vi "Measurement Logic Main.vi"(8 "error in":errorcluster, 9 "measurement configuration":T4={"SERIAL CHANNEL"="SI1", "PATH TO CONFIGURATION SCRIPT"="\"C:\\dev\\scripts\\Image Receiver Scripts\\9296A_RAW8.cpp\"", "REF. CLOCK  (Hz)"=25000000.0, "POC SOURCE"=0, "CSI-2 DATA SOURCE"=0, "SI ACTIVE LANE CNT"=4, "PAYLOAD DATA TYPE"=enum."RAW 8", "INTERPRETATION"=1, "VIRTUAL CHANNEL"=0, "PATTERN"=0, "ALGORITHM"=0, "RIO HANDLER"="PXI1Slot2", "AUTO. VISION DEVICE"=0, "SERIAL (SI) CHANNEL"=1, "BITFILE"="PXIe_1487_4_In_4_Out_Acq_Tap.lvbitx"} {"SERIAL (SI) CHANNEL" items=["SI0", "SI1"]; "AUTO. VISION DEVICE" items=["PXI1Slot2", "PXI1Slot5"]; "ALGORITHM" items=["BILINEAR", "VNG"]; "PATTERN" items=["GB", "GR", "BG", "RG"]; "INTERPRETATION" items=["Grayscale", "Bayer", "RGB", "YUV422", "YUV420", "Legacy YUV420"]; "SI ACTIVE LANE CNT" items=["1 LANE"=1, "2 LANE"=2, "4 LANE"=4]; "CSI-2 DATA SOURCE" items=["CORRECTED", "RAW"]; "POC SOURCE" items=["NONE", "INTERNAL", "AUXILIARY"]}, 10 "measure call context in":refnum<class "Measure Call Context.lvclass">, 11 "user event out":refnum<user-event>) -> (0 "Error Out":errorcluster, 2 "measure call context out":refnum<class "Measure Call Context.lvclass">, 3 "measurement results":T1 {"BYTES ACQUIRED" format="%#.6p"})   [LabVIEW 2025, in "Automotive Vision.lvclass"]
doc: "Contains the core logic for executing the measurement."
uses:
  Automotive Vision.lvclass
  <vilib>/Plug-In SDKs/Measurements/Measure Call Context/Measure Call Context.lvclass
  Measurement Configuration.ctl
  Measurement Results.ctl
  <instrlib>/FlexRIO/CSI-2/v2/Common/Types/LLP Data Type.ctl
  <vilib>/vision/Image Controls.llb/IMAQ Image.ctl
  <instrlib>/FlexRIO/API/Host/v1/NI FlexRIO/API/Wait for PoC Safe to Disconnect Channels Array.vi
  <vilib>/FPGAPlugInAG/Dynamic/niLvFpga_Close_Dynamic.vi
  <extravilib>/ChannelInstances/Event Messenger-bool/Instantiate.vi
  <vilib>/rvi/interface/nirviCloseFPGA/nirviCloseFPGA.xnode
  Automotive Vision.lvclass/Automotive Vision.ctl
  deps/NI148X/Getting Started/Host/Acq/GettingStarted_Acq_148X_Host.lvlib
  deps/NI148X/Getting Started/Host/Common/GettingStarted_Common_148X_Host.lvlib
  <instrlib>/FlexRIO/API/Host/v1/NI FlexRIO API v1.lvlib
  <instrlib>/FlexRIO/CSI-2/v2/Common/NI CSI-2 API Common v2.lvlib
panel:
  in  "Serial Channel (2nd Display)":fxp<+,3,3>
  in  "Serial Channel (1st Display)":fxp<+,3,3>
  in  "Acquired Serial Input Channel Data":T2(tab)
  out "Source Rate (fps)(1st Display)":dbl
  out "Update Rate (fps)(1st Display)":dbl
  out "1st channel display":T3(plugin-control)
  out "Bytes Acquired (1st Channel)":i64 format="%#.6p"
  out "Packets Logged (1st Channel)":i64
  out "Source Rate (fps)(2nd Display)":dbl
  out "Update Rate (fps)(2nd Display)":dbl
  out "2nd channel display":T3(plugin-control)
  out "Packets Logged (2nd Channel)":i64
  out "Bytes Acquired (2nd Channel)":i64 format="%#.6p"
  out "Acquisition In Progress":bool
  out "Acquisition Duration (s)":dbl format="%.1f"
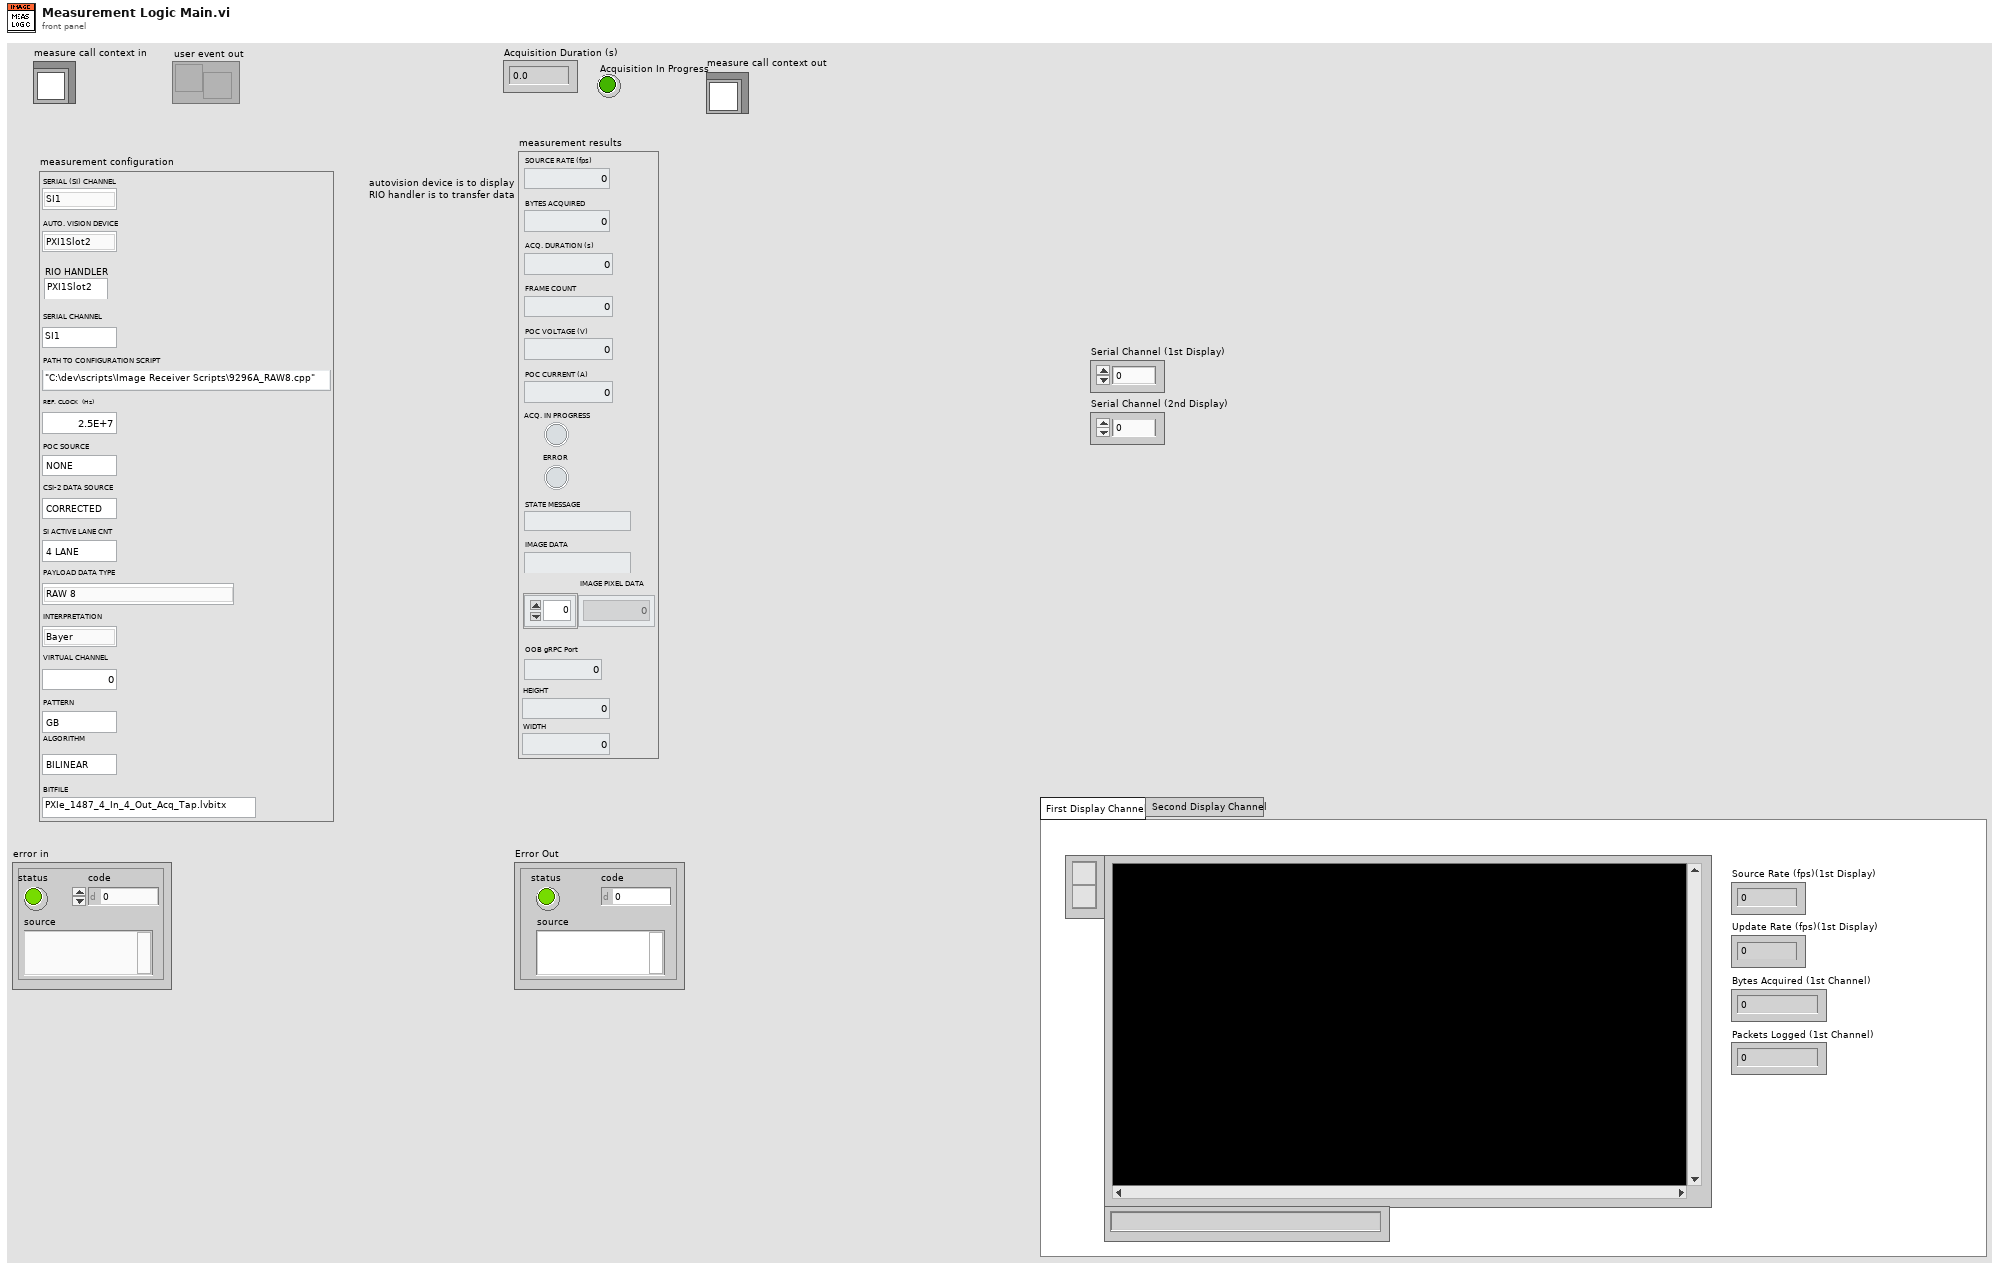
[diagram p1: front panel]
types:
  T1 = typedef "Automotive Vision.lvclass/Measurement Results.ctl" = cluster{"ACQ. IN PROGRESS":bool, "IMAGE PIXEL DATA":u32[], "ACQ. DURATION (s)":dbl, "SOURCE RATE (fps)":dbl, "BYTES ACQUIRED":u64, "FRAME COUNT":u64, "POC VOLTAGE (V)":dbl, "POC CURRENT (A)":dbl, "ERROR":bool, "STATE MESSAGE":string, "IMAGE DATA":string, "OOB gRPC Port":i32, "HEIGHT":u64, "WIDTH":u64}
  T2 = enum32{"First Display Channel", "Second Display Channel"}
  T3 = typedef "IMAQ Image.ctl" = refnum<image>
  T4 = typedef "Automotive Vision.lvclass/Measurement Configuration.ctl" = cluster{"SERIAL CHANNEL":string, "PATH TO CONFIGURATION SCRIPT":string, "REF. CLOCK  (Hz)":dbl, "POC SOURCE":u32, "CSI-2 DATA SOURCE":u32, "SI ACTIVE LANE CNT":u32, "PAYLOAD DATA TYPE":enum32{"Frame Start", "Frame End", "Line Start", "Line End", "End of Transmission", "Reserved 0", "Reserved 1", "Reserved 2", "Generic Short Packet 1", "Generic Short Packet 2", "Generic Short Packet 3", "Generic Short Packet 4", "Generic Short Packet 5", "Generic Short Packet 6", "Generic Short Packet 7", "Generic Short Packet 8", "Null", "Blanking Data", "Embedded 8-bit non Image Data", "Generic Long Packet 1", "Generic Long Packet 2", "Generic Long Packet 3", "Generic Long Packet 4", "Reserved 3", "YUV420 8-bit", "YUV420 10-bit", "Legacy YUV420 8-bit", "Reserved 4", "YUV420 8-bit Chroma Shifted", "YUV420 10-bit Chroma Shifted", "YUV422 8-bit", "YUV422 10-bit", "RGB444", "RGB555", "RGB565", "RGB666", "RGB888", "Reserved 5", "Reserved 6", "RAW 24", "RAW 6", "RAW 7", "RAW 8", "RAW 10", "RAW 12", "RAW 14", "RAW 16", "RAW 20", "User Defined 8-bit Data 1", "User Defined 8-bit Data 2", "User Defined 8-bit Data 3", "User Defined 8-bit Data 4", "User Defined 8-bit Data 5", "User Defined 8-bit Data 6", "User Defined 8-bit Data 7", "User Defined 8-bit Data 8", "USL Command", "Reserved 7", "Reserved 8", "Reserved 9", "Reserved 10", "Reserved 11", "Reserved 12", "LRTE EPD Spacer"}, "INTERPRETATION":u32, "VIRTUAL CHANNEL":u32, "PATTERN":u32, "ALGORITHM":u32, "RIO HANDLER":string, "AUTO. VISION DEVICE":u32, "SERIAL (SI) CHANNEL":u32, "BITFILE":string}
  T5 = typedef "NI CSI-2 API Common v2.lvlib/LLP Data Type.ctl" = enum8{"Frame Start", "Frame End", "Line Start", "Line End", "End of Transmission", "Reserved 0", "Reserved 1", "Reserved 2", "Generic Short Packet 1", "Generic Short Packet 2", "Generic Short Packet 3", "Generic Short Packet 4", "Generic Short Packet 5", "Generic Short Packet 6", "Generic Short Packet 7", "Generic Short Packet 8", "Null", "Blanking Data", "Embedded 8-bit non Image Data", "Generic Long Packet 1", "Generic Long Packet 2", "Generic Long Packet 3", "Generic Long Packet 4", "Reserved 3", "YUV420 8-bit", "YUV420 10-bit", "Legacy YUV420 8-bit", "Reserved 4", "YUV420 8-bit Chroma Shifted", "YUV420 10-bit Chroma Shifted", "YUV422 8-bit", "YUV422 10-bit", "RGB444", "RGB555", "RGB565", "RGB666", "RGB888", "Reserved 5", "Reserved 6", "RAW 24", "RAW 6", "RAW 7", "RAW 8", "RAW 10", "RAW 12", "RAW 14", "RAW 16", "RAW 20", "User Defined 8-bit Data 1", "User Defined 8-bit Data 2", "User Defined 8-bit Data 3", "User Defined 8-bit Data 4", "User Defined 8-bit Data 5", "User Defined 8-bit Data 6", "User Defined 8-bit Data 7", "User Defined 8-bit Data 8", "USL Command", "Reserved 7", "Reserved 8", "Reserved 9", "Reserved 10", "Reserved 11", "Reserved 12", "LRTE EPD Spacer"}
  T6 = typedef "GettingStarted_Common_148X_Host.lvlib/Serial Channel Configuration.ctl" = cluster{"Serial Channel":string, "FPGA Display Parameters":T7, "RAW Display Parameters":cluster{"Interpretation":T8, "Bayer Parameters":cluster{"Pattern":i32, "Algorithm":i32, "Red Gain":dbl, "Green Gain":dbl, "Blue Gain":dbl}}}
  T7 = typedef "NI CSI-2 API FPGA v2.lvlib/Display Parameters.ctl" = cluster{"virtual channel":fxp<+,4,4>, "payload data type":T5, "frame skip count":u16, "line skip count":u8, "pixel skip count":fxp<+,5,5>}
  T8 = typedef "GettingStarted_Common_148X_Host.lvlib/RAW Interpretation for Display.ctl" = enum16{"Grayscale", "Bayer", "RGB", "YUV422", "YUV420", "Legacy YUV420"}
  T9 = typedef "GettingStarted_Common_148X_Host.lvlib/Serial Channel Display Parameters.ctl" = cluster{"images":cluster{"grayscale":T3, "color":T3}, "RAW parameters":cluster{"interpretation":T8, "bayer parameters":cluster{"pattern":i32, "algorithm":i32, "red gain":dbl, "green gain":dbl, "blue gain":dbl}}}
  T10 = cluster{"Acquisition In Progress":refnum<vi>, "Acquisition Duration (s)":refnum<vi>, "Bytes Acquired (1st Channel)":refnum<vi>}
  T11 = typedef "Event Messenger-bool.lvlib/))Channel.ctl" = refnum<queue>
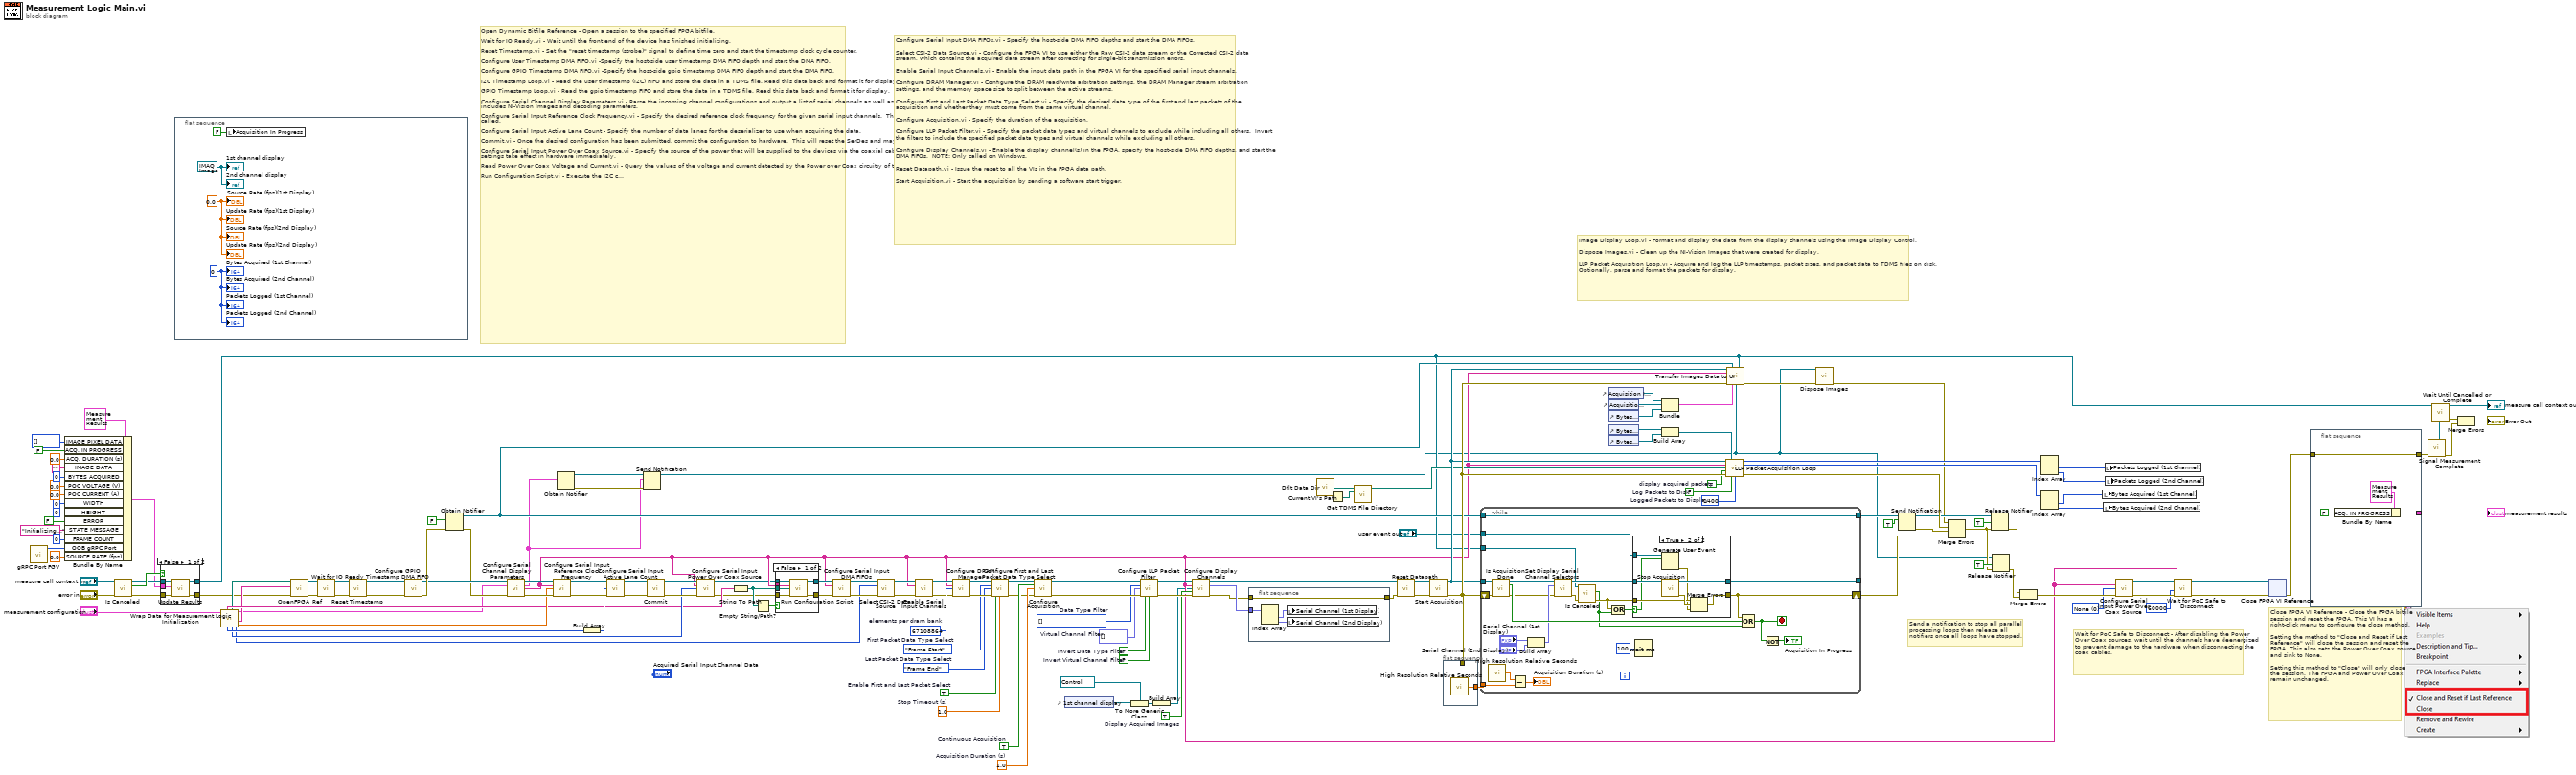
[diagram p0: block diagram]
diagram:
  w77 = i64 1400  # Logged Packets to Display
  w101 = FALSE  # Log Packets to Disk
  w131 = FALSE  # Invert Virtual Channel Filter
  w132 = FALSE  # Invert Data Type Filter
  w133 = fxp<+,4,4>[] []  # Virtual Channel Filter
  w97 = TRUE  # Display Acquired Images
  w135 = T5[] [] items=["Frame Start", "Frame End", "Line Start", "Line End", "End of Transmission", "Reserved 0", "Reserved 1", "Reserved 2", "Generic Short Packet 1", "Generic Short Packet 2", "Generic Short Packet 3", "Generic Short Packet 4", "Generic Short Packet 5", "Generic Short Packet 6", "Generic Short Packet 7", "Generic Short Packet 8", "Null", "Blanking Data", "Embedded 8-bit non Image Data", "Generic Long Packet 1", "Generic Long Packet 2", "Generic Long Packet 3", "Generic Long Packet 4", "Reserved 3", "YUV420 8-bit", "YUV420 10-bit", "Legacy YUV420 8-bit", "Reserved 4", "YUV420 8-bit Chroma Shifted", "YUV420 10-bit Chroma Shifted", "YUV422 8-bit", "YUV422 10-bit", "RGB444", "RGB555", "RGB565", "RGB666", "RGB888", "Reserved 5", "Reserved 6", "RAW 24", "RAW 6", "RAW 7", "RAW 8", "RAW 10", "RAW 12", "RAW 14", "RAW 16", "RAW 20", "User Defined 8-bit Data 1", "User Defined 8-bit Data 2", "User Defined 8-bit Data 3", "User Defined 8-bit Data 4", "User Defined 8-bit Data 5", "User Defined 8-bit Data 6", "User Defined 8-bit Data 7", "User Defined 8-bit Data 8", "USL Command", "Reserved 7", "Reserved 8", "Reserved 9", "Reserved 10", "Reserved 11", "Reserved 12", "LRTE EPD Spacer"]  # Data Type Filter
  w138 = 1.0  # Acquisition Duration (s)
  w141 = TRUE  # Continuous Acquisition
  w121 = 1.0  # Stop Timeout (s)
  w122 = TRUE  # Enable First and Last Packet Select
  w119 = LLP_Data_Type."Frame End"  # Last Packet Data Type Select
  w120 = LLP_Data_Type."Frame Start"  # First Packet Data Type Select
  w58 = 0 items=["None", "Internal", "Auxiliary"] ("power over coax source")
  w78 = TRUE  # display acquired packets
  w147 = u32 67108864  # elements per dram bank
  # "Wait for PoC Safe to Disconnect - After disabling the Power Over Coax sources, wait until the channels have deenergized to prevent damage to the hardware when disconnecting the coax cables."
  # "Send a notification to stop all parallel processing loops then release all notifiers once all loops have stopped."
  # "Image Display Loop.vi - Format and display the data from the display channels using the Image Display Control.   \n\nDispose Images.vi - Clean up the NI-Vision Images that were created for display.\n\nLLP Packet Acquisition Loop.vi - Acquire and log the LLP timestamps, packet sizes, and packet data to TDMS files on disk.  Optionally, parse and format the packets for display."
  # "Configure Serial Input DMA FIFOs.vi - Specify the host-side DMA FIFO depths and start the DMA FIFOs.\n\nSelect CSI-2 Data Source.vi - Configure the FPGA VI to use either the Raw CSI-2 data stream or the Corrected CSI-2 data stream, which contains the acquired data stream after correcting for single-bit transmission errors.\n\nEnable Serial Input Channels.vi - Enable the input data path in the FPGA VI for the specified serial input channels.\n\nConfigure DRAM Manager.vi - Configure the DRAM read/write arbitration settings, the DRAM Manager stream arbitration settings, and the memory space size to split between the active streams.\n\nConfigure First and Last Packet Data Type Select.vi - Specify the desired data type of the first and last packets of the acquisition and whether they must come from the same virtual channel.\n\nConfigure Acquisition.vi - Specify the duration of the acquisition.\n\nConfigure LLP Packet Filter.vi - Specify the packet data types and virtual channels to exclude while including all others.  Invert the filters to include the specified packet data types and virtual channels while excluding all others.\n\nConfigure Display Channels.vi - Enable the display channel(s) in the FPGA, specify the host-side DMA FIFO depths, and start the DMA FIFOs.  NOTE: Only called on Windows. \n\nReset Datapath.vi - Issue the reset to all the VIs in the FPGA data path.\n\nStart Acquisition.vi - Start the acquisition by sending a software start trigger."
  # "Close FPGA VI Reference - Close the FPGA bitfile session and reset the FPGA. This VI has a right-click menu to configure the close method. \n\nSetting the method to \"Close and Reset if Last Reference\" will close the session and reset the FPGA. This also sets the Power Over Coax source and sink to None.\n\nSetting this method to \"Close\" will only close the session. The FPGA and Power Over Coax remain unchanged."
  # "Open Dynamic Bitfile Reference - Open a session to the specified FPGA bitfile.\n\nWait for IO Ready.vi - Wait until the front end of the device has finished initializing.\n\nReset Timestamp.vi - Set the \"reset timestamp (strobe)\" signal to define time zero and start the timestamp clock cycle counter.\n\nConfigure User Timestamp DMA FIFO.vi -Specify the host-side user timestamp DMA FIFO depth and start the DMA FIFO.\n\nConfigure GPIO Timestamp DMA FIFO.vi -Specify the host-side gpio timestamp DMA FIFO depth and start the DMA FIFO.\n\nI2C Timestamp Loop.vi - Read the user timestamp (I2C) FIFO and store the data in a TDMS file. Read this data back and format it for display.\n\nGPIO Timestamp Loop.vi - Read the gpio timestamp FIFO and store the data in a TDMS file. Read this data back and format it for display.\n\nConfigure Serial Channel Display Parameters.vi - Parse the incoming channel configurations and output a list of serial channels as well as a list of serial channel display parameters, which includes NI-Vision Images and decoding parameters.\n\nConfigure Serial Input Reference Clock Frequency.vi - Specify the desired reference clock frequency for the given serial input channels.  These settings do not take effect until Commit.vi is called.\n\nConfigure Serial Input Active Lane Count - Specify the number of data lanes for the deserializer to use when acquiring the data. \n\nCommit.vi - Once the desired configuration has been submitted, commit the configuration to hardware.  This will reset the SerDes and may cause GPIO lines to toggle. \n\nConfigure Serial Input Power Over Coax Source.vi - Specify the source of the power that will be supplied to the devices via the coaxial cables attached to the given serial input channels.  These settings take effect in hardware immediately.\n\nRead Power Over Coax Voltage and Current.vi - Query the values of the voltage and current detected by the Power over Coax circuitry of the given serial channels.\n\nRun Configuration Script.vi - Execute the I2C commands in the specified script file for the given serial channels.  The script is used to configure the serializer, deserializer, or other I2C slave device, such as the image sensor."
  n1 = call "gRPC Port FGV.vi"() -> ("Listening Port out"=w28:i32)  [unwired: 11 in]
  n2 = Bundle By Name(cluster=T1 {"ACQ. IN PROGRESS"=FALSE, "IMAGE PIXEL DATA"=[], "ACQ. DURATION (s)"=0.0, "SOURCE RATE (fps)"=0.0, "BYTES ACQUIRED"=0, "FRAME COUNT"=0, "POC VOLTAGE (V)"=0.0, "POC CURRENT (A)"=0.0, "ERROR"=FALSE, "STATE MESSAGE"="", "IMAGE DATA"="", "OOB gRPC Port"=0, "HEIGHT"=0, "WIDTH"=0} ("Measurement Results"), "IMAGE PIXEL DATA"=u32[] [], "ACQ. IN PROGRESS"=FALSE, "ACQ. DURATION (s)"=0.0, "IMAGE DATA"="", "BYTES ACQUIRED"=u64 0, "POC VOLTAGE (V)"=0.0, "POC CURRENT (A)"=0.0, "WIDTH"=u64 0, "HEIGHT"=u64 0, "ERROR"=FALSE, "STATE MESSAGE"="Initializing...", "FRAME COUNT"=u64 0, "OOB gRPC Port"=w28, "SOURCE RATE (fps)"=0.0) -> (w24:T1)
  n3 = call <vilib>:"Is Canceled.vi"("error in"="error in", "measure call context in"="measure call context in") -> ("error out"=w27:errorcluster, "is canceled?"=w26:bool, "measure call context out"=w25:refnum<class "Measure Call Context.lvclass">)  [unwired: 7 in]
  n4 = case shown="False" w26 {
    tunnel: w24 -> [w156 _]
    tunnel: [w155 w158] -> w21
    tunnel: w25 -> [w154 w157]
    tunnel: w27 -> [w153 w158]
    tunnel: [w152 w157] -> w6
    frame False {
      n5 = call <vilib>:"Update Results.vi"("error in"=w153, "measurement results"=w156, "measure call context in"=w154) -> ("error out"=w155:errorcluster, "measure call context out"=w152:refnum<class "Measure Call Context.lvclass">)  [unwired: 7 in]
    }
    frame True {
    }
  }
  n6 = flat-sequence {
    frame #0 {
      w160 = i64 0 ("Number of Packets Acquired (1st Channel)")
      w161 = 0.0 ("display fps (2nd display)")
      w162 = T3 refnum ("first channel display")
      n7 = local write "Acquisition In Progress"(FALSE ("Acquisition In Progress")) -> ()
      "1st channel display" <- w162
      "2nd channel display" <- w162
      "Update Rate (fps)(1st Display)" <- w161
      "Update Rate (fps)(2nd Display)" <- w161
      "Packets Logged (1st Channel)" <- w160
      "Packets Logged (2nd Channel)" <- w160
      "Source Rate (fps)(1st Display)" <- w161
      "Source Rate (fps)(2nd Display)" <- w161
      "Bytes Acquired (1st Channel)" <- w160
      "Bytes Acquired (2nd Channel)" <- w160
    }
  }
  n8 = call "Wrap Data for Measurement Logic Initialization.vi"("measurement configuration"="measurement configuration") -> ("REF. CLOCK  (Hz)"=w47:dbl, "RIO HANDLER"=w43:string, "CSI-2 DATA SOURCE"=w48:u32, "Serial Input Configuration"=w36:T6[], "POC SOURCE"=w49:u32, "appended path"=w42:path, "SI ACTIVE LANE CNT"=w50:u32, "PATH TO CONFIGURATION SCRIPT"=w46:string)  [unwired: 3 in]
  n9 = call "OpenFPGA_Ref.vi"("error in"=w21, "RIO HANDLER"=w43, "Bitfile path"=w42) -> ("error out"=w37:errorcluster, "Refnum out"=w134:refnum<k20>)  [unwired: 7 in]
  n10 = call <instrlib>:"Wait for IO Ready.vi"("fpga interface in"=w134, "error in"=w37) -> ("fpga interface out"=w94:refnum<k20>, "error out"=w95:errorcluster)  [unwired: 10 in, 2 out]
  n11 = call "Reset Timestamp.vi"("fpga interface in"=w94, "error in (no error)"=w95) -> ("fpga interface out"=w2:refnum<k20>, "error out"=w1:errorcluster)  [unwired: 12 in]
  n12 = call "Configure GPIO Timestamp DMA FIFO.vi"("fpga interface in"=w2, "error in (no error)"=w1) -> ("fpga interface out"=w82:refnum<k20>, "error out"=w84:errorcluster)  [unwired: 12 in]
  n13 = Obtain Notifier(notification data type=FALSE ("result"), error in (no error)=w84) -> (notifier out=w70:refnum<notifier>, error out=w81:errorcluster)  [unwired: 2 in, 1 out]
  n14 = call "Configure Serial Channel Display Parameters.vi"("fpga interface in"=w82, "serial channel configurations"=w36, "error in (no error)"=w81) -> ("fpga interface out"=w111:refnum<k20>, "serial channel display parameters"=w67:T9[], "serial channels"=w35:string[], "error out"=w110:errorcluster)  [unwired: 9 in]
  n15 = call "Configure Serial Input Reference Clock Frequency.vi"("fpga interface in"=w111, "serial input channels"=w35, "serial input reference clock frequency (Hz)"=w47, "error in (no error)"=w110) -> ("fpga interface out"=w75:refnum<k20>, "error out"=w74:errorcluster)  [unwired: 10 in]
  n16 = Obtain Notifier(notification data type=w67) -> (notifier out=w69:refnum<notifier>, error out=w68:errorcluster)  [unwired: 3 in, 1 out]
  n17 = Build Array(w50) -> (w71:u32[])
  n18 = call "Configure Serial Input Active Lane Count.vi"("fpga interface in"=w75, "serial input active lane counts"=w71, "error in (no error)"=w74) -> ("fpga interface out"=w73:refnum<k20>, "error out"=w72:errorcluster)  [unwired: 11 in]
  n19 = Send Notification(notification=w67, notifier=w69, error in (no error)=w68) -> (notifier out=w5:refnum<notifier>)  [unwired: 1 out]
  n20 = call <instrlib>:"Commit.vi"("fpga interface in"=w73, "error in"=w72) -> ("fpga interface out"=w136:refnum<k20>, "error out"=w137:errorcluster)  [unwired: 12 in]
  n21 = call "Configure Serial Input Power Over Coax Source.vi"("fpga interface in"=w136, "serial input channels"=w35, "power over coax source"=w49, "error in (no error)"=w137) -> ("fpga interface out"=w30:refnum<k20>, "error out"=w29:errorcluster)  [unwired: 9 in, 1 out]
  n22 = String To Path(string=w46) -> (path=w45:path)
  n23 = Empty String/Path?(string/path=w45) -> (empty?=w96:bool)
  n24 = case shown="False" w96 {
    tunnel: [w168 w169] -> w145
    tunnel: [w167 w170] -> w140
    tunnel: w29 -> [w166 w169]
    tunnel: w30 -> [w165 w170]
    tunnel: w35 -> [w164 _]
    tunnel: w45 -> [w163 _]
    frame False {
      n25 = call "Run Configuration Script.vi"("fpga interface in"=w165, "serial channels"=w164, "configuration script"=w163, "error in (no error)"=w166) -> ("fpga interface out"=w167:refnum<k20>, "error out"=w168:errorcluster)  [unwired: 10 in]
    }
    frame True {
    }
  }
  n26 = call "Configure Serial Input DMA FIFOs.vi"("fpga interface in"=w140, "serial channels"=w35, "error in (no error)"=w145) -> ("fpga interface out"=w130:refnum<k20>, "error out"=w127:errorcluster)  [unwired: 11 in]
  n27 = call "Select CSI-2 Data Source.vi"("fpga interface in"=w130, "csi-2 data source"=w48, "error in (no error)"=w127) -> ("fpga interface out"=w129:refnum<k20>, "error out"=w128:errorcluster)  [unwired: 11 in]
  n28 = call "Enable Serial Input Channels.vi"("fpga interface in"=w129, "serial input channels"=w35, "error in (no error)"=w128) -> ("fpga interface out"=w139:refnum<k20>, "error out"=w146:errorcluster)  [unwired: 11 in]
  n29 = call "Configure DRAM Manager.vi"("fpga interface in"=w139, "serial channels"=w35, "elements per dram bank"=w147, "error in (no error)"=w146) -> ("fpga interface out"=w123:refnum<k20>, "error out"=w126:errorcluster)  [unwired: 10 in]
  n30 = call "Configure First and Last Packet Data Type Select.vi"("fpga interface in"=w123, "first packet data type select"=w120, "last packet data type select"=w119, "error in (no error)"=w126, "enable first and last packet select"=w122, "stop timeout (s)"=w121) -> ("fpga interface out"=w124:refnum<k20>, "error out"=w125:errorcluster)  [unwired: 8 in]
  n31 = call "Configure Acquisition.vi"("fpga interface in"=w124, "continuous acquisition (T)"=w141, "acquisition duration (s)"=w138, "error in (no error)"=w125) -> ("fpga interface out"=w142:refnum<k20>, "error out"=w143:errorcluster)  [unwired: 10 in]
  n32 = control-ref of="1st channel display"() -> (w32:refnum<vi>)
  n33 = To More Generic Class(target class=refnum<vi> refnum ("image display reference"), reference=w32) -> (generic class reference=w34:refnum<vi>)
  n34 = call "Configure LLP Packet Filter.vi"("fpga interface in"=w142, "data type filter"=w135, "virtual channel filter"=w133, "error in (no error)"=w143, "invert data type filter"=w132, "invert virtual channel filter"=w131) -> ("fpga interface out"=w112:refnum<k20>, "error out"=w109:errorcluster)  [unwired: 8 in]
  n35 = Build Array(w34) -> (w31:refnum<vi>[])
  n36 = call "Configure Display Channels.vi"("fpga interface in"=w112, "serial channels"=w35, "display references in"=w31, "enable image display"=w97, "error in (no error)"=w109) -> ("fpga interface out"=w108:refnum<k20>, "display serial channels"=w107:fxp<+,3,3>[], "error out"=w106:errorcluster)  [unwired: 7 in, 1 out]
  n37 = flat-sequence {
    tunnel: w107 -> [w172]
    tunnel: w106 -> [w171]
    tunnel: [w171] -> w105
    frame #0 {
      n38 = Index Array(array=w172) -> (element #1=w174:fxp<+,3,3>, element #2=w173:fxp<+,3,3>)  [unwired: 2 in]
      n39 = local write "Serial Channel (1st Display)"(w174) -> ()
      n40 = local write "Serial Channel (2nd Display)"(w173) -> ()
    }
  }
  n41 = call <vilib>:"Dflt Data Dir.vi"() -> ("App:Default Data Directory"=w44:path)
  n42 = Current VI's Path() -> (path=w115:path)
  n43 = call "Get TDMS File Directory.vi"("tdms file directory in"=w44, "calling vi path"=w115) -> ("tdms file directory out"=w80:path)  [unwired: 13 in]
  n44 = call "Reset Datapath.vi"("fpga interface in"=w108, "error in (no error)"=w105) -> ("fpga interface out"=w144:refnum<k20>, "error out"=w83:errorcluster)  [unwired: 12 in]
  n45 = call "Start Acquisition.vi"("fpga interface in"=w144, "error in (no error)"=w83) -> ("fpga interface out"=w92:refnum<k20>, "error out"=w93:errorcluster)  [unwired: 12 in]
  n46 = flat-sequence {
    tunnel: [w175] -> w116
    tunnel: w93 -> [_]
    frame #0 {
      n47 = call <vilib>:"High Resolution Relative Seconds.vi"() -> ("relative seconds"=w175:dbl)
    }
  }
  n48 = while {
    shift-right: [w179] -> w76
    shift-left: w93 -> [w190]
    tunnel: w92 -> [w192]
    tunnel: w116 -> [w196]
    tunnel: w70 -> [w189]
    tunnel: [w189] -> w89
    tunnel: [w180] -> w62
    tunnel: w6 -> [w186]
    tunnel: "user event out" -> [w176]
    stop <- w191 stop-if-true
    n49 = call <vilib>:"High Resolution Relative Seconds.vi"() -> ("relative seconds"=w197:dbl)
    n50 = call "Is Acquisition Done.vi"("fpga interface in"=w192, "error in (no error)"=w190) -> ("fpga interface out"=w182:refnum<k20>, "acquisition done"=w199:bool, "error out"=w181:errorcluster)  [unwired: 11 in]
    n51 = Subtract(x=w197, y=w196) -> (x-y=→"Acquisition Duration (s)":dbl)
    n52 = Build Array("Serial Channel (1st Display)", "Serial Channel (2nd Display)") -> (w193:fxp<+,3,3>[])
    n53 = call "Set Display Serial Channel Selectors.vi"("fpga interface in"=w182, "display serial channel selectors"=w193, "error in (no error)"=w181) -> ("fpga interface out"=w187:refnum<k20>, "error out"=w188:errorcluster)  [unwired: 11 in]
    n54 = call <vilib>:"Is Canceled.vi"("error in"=w188, "measure call context in"=w186) -> ("error out"=w184:errorcluster, "is canceled?"=w178:bool)  [unwired: 7 in, 1 out]
    n55 = Compound Arithmetic op=OR(w184, w178) -> (w177:bool)
    n56 = case shown="True" w177 {
      selector: w177 -> [_ w203]
      tunnel: [w201 w206] -> w179
      tunnel: w184 -> [w201 w205]
      tunnel: [w200 w208] -> w180
      tunnel: w187 -> [w200 w207]
      tunnel: w176 -> [_ w204]
      frame False {
      }
      frame True {
        n57 = Generate User Event(user event=w204, event data cluster=w203) -> (error out=w202:errorcluster)  [unwired: 2 in, 1 out]
        n58 = call "Stop Acquisition.vi"("fpga interface in"=w207) -> ("fpga interface out"=w208:refnum<k20>, "error out"=w209:errorcluster)  [unwired: 13 in]
        n59 = Merge Errors(w205, w209, w202) -> (w206:errorcluster)
      }
    }
    n60 = Wait (ms)(milliseconds to wait=u32 100) -> ()  [unwired: 1 out]
    n61 = Compound Arithmetic op=OR(w179, w199, w178) -> (w191:bool)
    n62 = Not(x=w191) -> (.not. x?=→"Acquisition In Progress":bool)
  }
  n63 = control-ref of="Acquisition In Progress"() -> (w41:refnum<vi>)
  n64 = control-ref of="Acquisition Duration (s)"() -> (w40:refnum<vi>)
  n65 = control-ref of="Bytes Acquired (1st Channel)"() -> (w39:refnum<vi>)
  n66 = control-ref of="Bytes Acquired (1st Channel)"() -> (w118:refnum<vi>)
  n67 = control-ref of="Bytes Acquired (2nd Channel)"() -> (w117:refnum<vi>)
  n68 = Bundle("Acquisition In Progress"=w41, "Acquisition Duration (s)"=w40, "Bytes Acquired (1st Channel)"=w39) -> (w38:T10)  [unwired: 1 in]
  n69 = Build Array(w118, w117) -> (w114:refnum<vi>[])
  n70 = call "LLP Packet Acquisition Loop.vi"("fpga interface in"=w92, "bytes acquired references"=w114, "Serial Channels"=w35, "tdms file directory"=w80, "display acquired packets"=w78, "error in"=w93, "log to disk"=w101, "num packets to read"=w77) -> ("number of packets acquired"=w113:i64[], "number of bytes acquired"=w100:i64[], "error out"=w90:errorcluster)  [unwired: 4 in, 1 out]
  n71 = call "Transfer Images Data to UI.vi"("fpga interface in"=w92, "'stop' notifier"=w70, "measure call context in"=w6, "Active Channel"=w35, "error in"=w93, "References"=w38, "raw display notifier"=w5) -> ("error out"=w102:errorcluster)  [unwired: 7 in, 1 out]
  n72 = call "Dispose Images.vi"("raw display notifier"=w5, "error in (no error)"=w102) -> ("error out"=w79:errorcluster)  [unwired: 13 in]
  n73 = Send Notification(notification=TRUE, notifier=w89) -> (notifier out=w88:refnum<notifier>, error out=w87:errorcluster)  [unwired: 1 in]
  n74 = Merge Errors(w79, w90, w87, w76) -> (w65:errorcluster)
  n75 = Release Notifier(notifier=w88, force destroy? (F)=TRUE, error in (no error)=w65) -> (error out=w64:errorcluster)  [unwired: 2 out]
  n76 = Release Notifier(notifier=w5, force destroy? (F)=TRUE, error in (no error)=w65) -> (error out=w63:errorcluster)  [unwired: 2 out]
  n77 = Merge Errors(w64, w63) -> (w61:errorcluster)
  n78 = Index Array(array=w113) -> (element #1=w104:i64, element #2=w103:i64)  [unwired: 2 in]
  n79 = Index Array(array=w100) -> (element #1=w99:i64, element #2=w98:i64)  [unwired: 2 in]
  n80 = local write "Bytes Acquired (1st Channel)"(w99) -> ()
  n81 = local write "Bytes Acquired (2nd Channel)"(w98) -> ()
  n82 = local write "Packets Logged (1st Channel)"(w104) -> ()
  n83 = local write "Packets Logged (2nd Channel)"(w103) -> ()
  n84 = call "Configure Serial Input Power Over Coax Source.vi"("fpga interface in"=w62, "serial input channels"=w35, "power over coax source"=w58, "error in (no error)"=w61) -> ("fpga interface out"=w56:refnum<k20>, "error out"=w57:errorcluster)  [unwired: 9 in, 1 out]
  n85 = call-poly <instrlib>:"Wait for PoC Safe to Disconnect.vi"("error in"=w57, "Timeout (ms)"=60000 ("Wait for Safe to Disconnect Timeout (ms)"), "Channels"=w35, "fpga interface in"=w56) -> ("error out"=w60:errorcluster, "fpga interface out"=w59:refnum<k20>)  [unwired: 6 in]
  n86 = xnode ("Close FPGA VI Reference")("FPGA VI Reference In"=w59, "error in"=w60) -> ("error out"=w52:errorcluster)
  n87 = flat-sequence {
    tunnel: [w212] -> w53
    tunnel: w52 -> [w210]
    tunnel: [w210] -> w4
    frame #0 {
      n88 = Bundle By Name(cluster=T1 {"ACQ. IN PROGRESS"=FALSE, "IMAGE PIXEL DATA"=[], "ACQ. DURATION (s)"=0.0, "SOURCE RATE (fps)"=0.0, "BYTES ACQUIRED"=0, "FRAME COUNT"=0, "POC VOLTAGE (V)"=0.0, "POC CURRENT (A)"=0.0, "ERROR"=FALSE, "STATE MESSAGE"="", "IMAGE DATA"="", "OOB gRPC Port"=0, "HEIGHT"=0, "WIDTH"=0} ("Measurement Results"), "ACQ. IN PROGRESS"=FALSE) -> (w212:T1)
    }
  }
  n89 = call "Signal Measurement Complete.vi"("error in (no error)"=w4) -> ("error out"=w149:errorcluster, "done channel"=w150:T11)  [unwired: 9 in]
  n90 = call "Wait Until Cancelled or Complete.vi"("done channel"=w150, "measure call context in"=w6) -> ("error out"=w148:errorcluster, "measure call context out"=→"measure call context out":refnum<class "Measure Call Context.lvclass">)  [unwired: 8 in]
  n91 = Merge Errors(w148, w149) -> (→"Error Out":errorcluster)
  "measurement results" <- w53
